vi "read_P_Gas.vi"() -> (0 "H2 Flush":bool, 1 "P Gas Actual Flow Rate":dbl, 2 "Remote":bool, 3 "Run":bool, 4 "Gas In":bool, 5 "Active":bool)   [LabVIEW 2011]
uses:
  low_level_proc/globals.vi
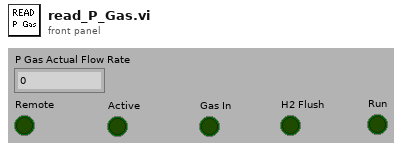
[diagram p1: front panel]
types:
  T1 = typedef "relaySpec.ctl" = cluster{"Card Index":u16, "Relay Index":u16}
  T2 = typedef "DA_Spec.ctl" = cluster{"Card Index":u16, "Channel Index":u16}
  T3 = typedef "AD_Spec.ctl" = u16
  T4 = cluster{"Relay Functions":cluster{"Remote":T1, "Active":T1, "Gas in":T1, "H2 flush":T1, "Run":T1}, "D/A Functions":cluster{"Flow":T2}, "Flow Range":cluster{"Flow (PGMFC1)":u16}, "A/D Functions":cluster{"Flow":T3}}
  T5 = cluster{"Remote":T1, "Active":T1, "Gas in":T1, "H2 flush":T1, "Run":T1}
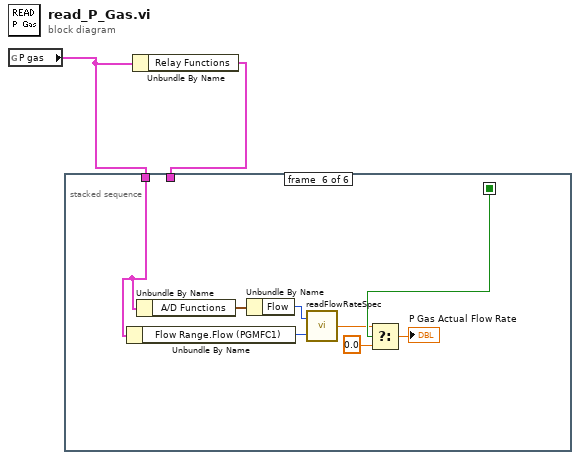
[diagram p0: block diagram]
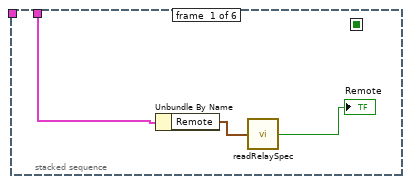
[diagram p2: hidden frame]
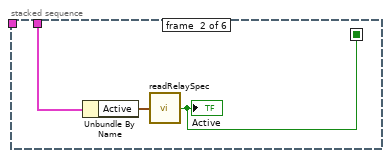
[diagram p3: hidden frame]
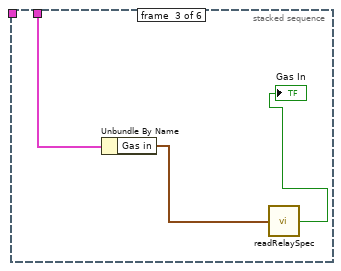
[diagram p4: hidden frame]
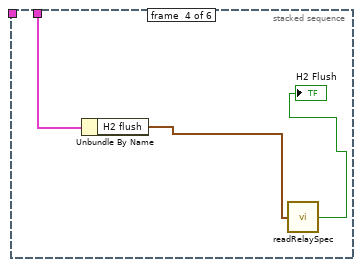
[diagram p5: hidden frame]
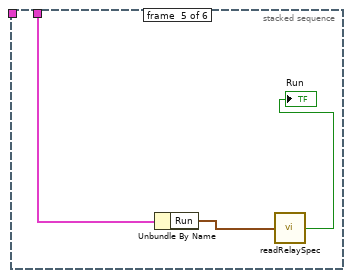
[diagram p6: hidden frame]
diagram:
  n1 = global read "globals.vi" "P gas"() -> (w2:T4)
  n2 = Unbundle By Name(w2) -> ("Relay Functions"=w1:T5)
  n3 = stacked-sequence {
    seq-local: [_ w8 _ _ _ _] -> [_ _ _ _ _ w25]
    tunnel: w1 -> [w3 w6 w9 w12 w15 _]
    tunnel: w2 -> [_ _ _ _ _ w19]
    frame #0 {
      n4 = Unbundle By Name(w3) -> ("Remote"=w4:T1)
      n5 = call "readRelaySpec.vi"("RelaySpec"=w4) -> ("Relay Status"=→"Remote":bool)
    }
    frame #1 {
      n6 = Unbundle By Name(w6) -> ("Active"=w7:T1)
      n7 = call "readRelaySpec.vi"("RelaySpec"=w7) -> ("Relay Status"=w8:bool)
      "Active" <- w8
    }
    frame #2 {
      n8 = Unbundle By Name(w9) -> ("Gas in"=w10:T1)
      n9 = call "readRelaySpec.vi"("RelaySpec"=w10) -> ("Relay Status"=→"Gas In":bool)
    }
    frame #3 {
      n10 = Unbundle By Name(w12) -> ("H2 flush"=w13:T1)
      n11 = call "readRelaySpec.vi"("RelaySpec"=w13) -> ("Relay Status"=→"H2 Flush":bool)
    }
    frame #4 {
      n12 = Unbundle By Name(w15) -> ("Run"=w16:T1)
      n13 = call "readRelaySpec.vi"("RelaySpec"=w16) -> ("Relay Status"=→"Run":bool)
    }
    frame #5 {
      n14 = Unbundle By Name(w19) -> ("Flow Range.Flow (PGMFC1)"=w18:u16)
      n15 = Unbundle By Name(w19) -> ("A/D Functions"=w20:cluster{"Flow":T3})
      n16 = Unbundle By Name(w20) -> ("Flow"=w21:T3)
      n17 = call "readFlowRateSpec.vi"("Flow range Index"=w18, "Channel Index"=w21) -> ("Flow Rate (sccm)"=w22:dbl)
      n18 = Select(t=w22, s=w25, f=0.0) -> (s? t:f=→"P Gas Actual Flow Rate":dbl)
    }
  }
